vi "CRDS Server.vi"(10 "nCRD in":refnum<class "nCRD.lvclass">, 11 "DVR In":refnum<data-value>) -> (3 "nCRD out":refnum<class "nCRD.lvclass">)   [LabVIEW 2015]
uses:
  Data/Nicholas Data.lvclass
  CRD/nCRD.lvclass
  Reusable/Instrument/state.ctl
  Reusable/Session Log/System Log.lvclass
  Reusable/Session APIs/File Access/Config Data/Config Data.lvclass
  Reusable/Session Log/System Log.lvclass/System Log.ctl
  Reusable/Session APIs/File Access/Config Data/Config Data.lvclass/Config Data.ctl
  Reusable/Instrument/Instrument.lvclass/Instrument.ctl
  CRD/nCRD.lvclass/nCRD.ctl
  Reusable/Session APIs/File Access/Config Data/Accessors/Write Cfg Path.vi
  Reusable/Session Log/Accessors/Write Main Path.vi
  Reusable/Instrument/Write Log Session.vi
  Reusable/Instrument/Write Cfg Session.vi
  Reusable/Instrument/Instrument.lvclass
  <userlib>/_Session Fwk/Session - Root.lvclass
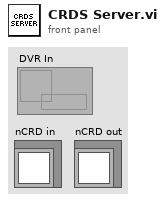
[diagram p1: front panel]
types:
  T1 = typedef "Instrument.lvclass/state.ctl" = enum8{"Configure", "Acquire", "Wait", "Quit", "Handle Error", "NOOP"}
  T2 = typedef "Session - Root.lvclass/Session Handle.ctl" = refnum<data-value>
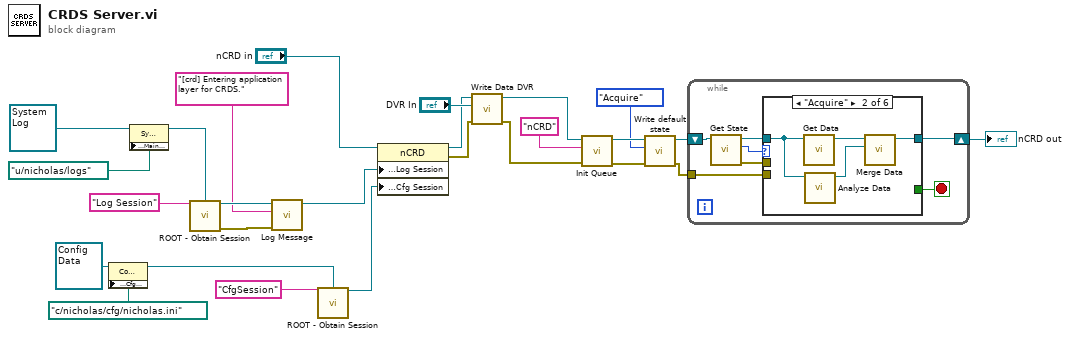
[diagram p0: block diagram]
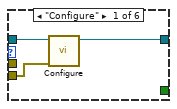
[diagram p2: hidden frame]
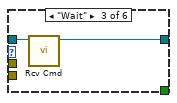
[diagram p3: hidden frame]
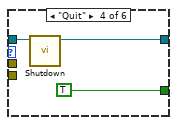
[diagram p4: hidden frame]
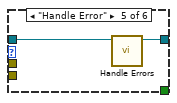
[diagram p5: hidden frame]
diagram:
  n1 = property class="Config Data"(reference=refnum<class "Config Data.lvclass"> refnum ("Config Data"), "Accessors:Cfg Path"=path "c:/nicholas/cfg/nicholas.ini" ("Cfg Path")) -> (reference out=w6:refnum<class "Config Data.lvclass">)  [unwired: 1 in, 1 out]
  n2 = property class="Sys Log"(reference=refnum<class "System Log.lvclass"> refnum ("Sys Log"), "Accessors:Main Path"=path "u:/nicholas/logs" ("Main Path")) -> (reference out=w14:refnum<class "System Log.lvclass">)  [unwired: 1 in, 1 out]
  n3 = call <userlib>:"ROOT - Obtain Session.vi"("Session Name ()"="Log Session", "OBJ - Session"=w14) -> ("Session Handle"=w11:T2, "error out"=w10:errorcluster)  [unwired: 11 in, 1 out]
  n4 = call "Log Message.vi"("error in"=w10, "MSG In"="[crd] Entering application layer for CRDS.", "session in"=w11) -> ("session out"=w8:T2)  [unwired: 7 in, 1 out]
  n5 = call <userlib>:"ROOT - Obtain Session.vi"("Session Name ()"="CfgSession", "OBJ - Session"=w6) -> ("Session Handle"=w3:T2)  [unwired: 11 in, 2 out]
  n6 = property class="nCRD"(reference="nCRD in", "Accessors:Log Session"=w8, "Accessors:Cfg Session"=w3) -> (reference out=w12:refnum<class "nCRD.lvclass">, error out=w2:errorcluster)  [unwired: 1 in]
  n7 = call "Write Data DVR.vi"("error in (no error)"=w2, "Data DVR"="DVR In", "nCRD in"=w12) -> ("error out"=w17:errorcluster, "nCRD out"=w26:refnum<class "nCRD.lvclass">)  [unwired: 7 in]
  n8 = call "Init Queue.vi"("error in"=w17, "queue_name"="nCRD", "Instrument in"=w26) -> ("error out"=w24:errorcluster, "Instrument out"=w23:refnum<class "nCRD.lvclass">)  [unwired: 7 in]
  n9 = call "Write default state.vi"("error in (no error)"=w24, "instr state"=state."Acquire", "Instrument in"=w23) -> ("error out"=w22:errorcluster, "Instrument out"=w21:refnum<class "nCRD.lvclass">)  [unwired: 7 in]
  n10 = while {
    shift-right: [w29] -> w18
    shift-left: w21 -> [w30]
    tunnel: w22 -> [w28]
    stop <- w32 stop-if-true
    n11 = call "Get State.vi"("Instrument in"=w30) -> ("error out"=w27:errorcluster, "default state"=w33:T1, "Instrument out"=w31:refnum<class "nCRD.lvclass">)  [unwired: 8 in]
    n12 = case shown="\"Acquire\"" w33 {
      tunnel: [_ _ _ TRUE _ _] -> w32
      tunnel: w31 -> [w36 w40 w42 w44 w47 w48]
      tunnel: [w35 w39 w41 w43 w46 w48] -> w29
      tunnel: w28 -> [w34 _ _ _ _ _]
      tunnel: w27 -> [_ _ _ _ _ _]
      frame "Configure" {
        n13 = call-dynamic "Configure.vi"("error in"=w34, "nCRD in"=w36) -> ("nCRD out"=w35:refnum<class "nCRD.lvclass">)  [unwired: 8 in, 1 out]
      }
      frame "Acquire" {
        n14 = call-dynamic "Get Data.vi"("nCRD in"=w40) -> ("nCRD out"=w38:refnum<class "nCRD.lvclass">)  [unwired: 9 in, 1 out]
        n15 = call-dynamic "Analyze Data.vi"("nCRD in"=w40) -> ("nCRD out"=w37:refnum<class "nCRD.lvclass">)  [unwired: 9 in, 1 out]
        n16 = call-dynamic "Merge Data.vi"("Analyzed"=w37, "Acquired"=w38) -> ("CRDS out"=w39:refnum<class "nCRD.lvclass">)  [unwired: 8 in, 1 out]
      }
      frame "Wait" {
        n17 = call-dynamic "Rcv Cmd.vi"("nCRD in"=w42) -> ("nCRD out"=w41:refnum<class "nCRD.lvclass">)  [unwired: 9 in, 1 out]
      }
      frame "Quit" {
        n18 = call-dynamic "Shutdown.vi"("nCRD in"=w44) -> ("nCRD out"=w43:refnum<class "nCRD.lvclass">)  [unwired: 9 in, 1 out]
      }
      frame "Handle Error" {
        n19 = call-dynamic "Handle Errors.vi"("nCRD in"=w47) -> ("nCRD out"=w46:refnum<class "nCRD.lvclass">)  [unwired: 8 in, 2 out]
      }
      frame "NOOP", Default {
      }
    }
  }
  "nCRD out" <- w18
